vi "tcp shot server send data.vi"(8 "error in (no error)":errorcluster, 10 "Data in":T3, 11 "TCP Network Connection in":refnum<k5>) -> (0 "error out":errorcluster, 3 "TCP Network Connection out":refnum<k5>)   [LabVIEW 2020]
uses:
  tcp shot sender queue.ctl
  TCP Multiple Connections State.ctl
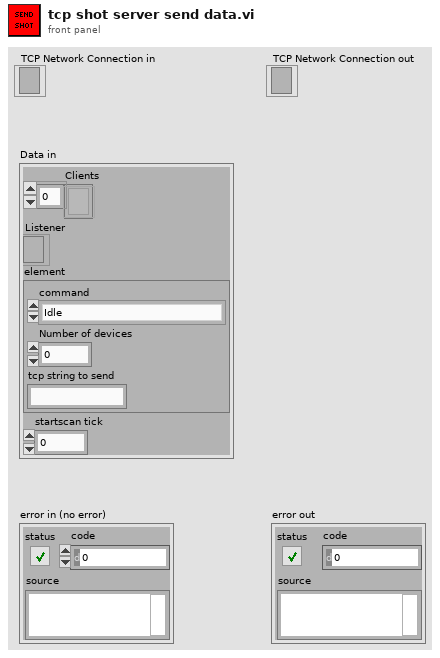
[diagram p1: front panel]
types:
  T1 = typedef "tcp shot sender queue.ctl" = cluster{"command":T2, "Number of devices":i32, "tcp string to send":string}
  T2 = typedef "TCP Multiple Connections State.ctl" = enum16{"Idle", "Initialize", "Start Scan", "Send Data", "Stop", "End Scan"}
  T3 = cluster{"Clients":refnum<k5>[], "Listener":refnum<k5>, "element":T1, "startscan tick":u32}
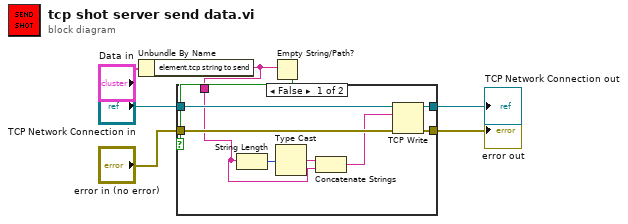
[diagram p0: block diagram]
diagram:
  n1 = Unbundle By Name("Data in") -> ("element.tcp string to send"=w6:string)
  n2 = Empty String/Path?(string/path=w6) -> (empty?=w7:bool)
  n3 = case shown="False" w7 {
    tunnel: [w15 w17] -> w1
    tunnel: "TCP Network Connection in" -> [w14 w16]
    tunnel: [w13 w16] -> w3
    tunnel: "error in (no error)" -> [w12 w17]
    tunnel: w6 -> [w8 _]
    frame False {
      n4 = String Length(string=w8) -> (length=w10:i32)
      n5 = Type Cast(x=w10) -> (*(type *) &x=w11:string)  [unwired: 1 in]
      n6 = Concatenate Strings(w11, w8) -> (w9:string)
      n7 = TCP Write(connection ID=w14, data in=w9, error in (no error)=w12) -> (connection ID out=w13:refnum<k5>, error out=w15:errorcluster)  [unwired: 2 out]
    }
    frame True {
    }
  }
  "TCP Network Connection out" <- w3
  "error out" <- w1
